vi "TWM Client Cmd Define Multiplexer Sequence.vi"(5 "timeout [ms]":i32=5000, 7 "end of packet key":string="TWM:command:EndOfPacket", 8 "error in":errorcluster, 10 "sequence item strings":string[](array[string]), 11 "handle":i32) -> (0 "error out":errorcluster, 3 "handle out":i32)   [LabVIEW 2020, in "TWM Client.lvlib"]
doc: "This will define multiplexer sequence. It's equivalent to manual setup in multiplexer panel. Sequence tag names must exist for currently selected multiplexer!"
uses:
  TWM Client.lvlib
  octave/infolib/1D String.vi
  octave/infolib/infolib.lvlib
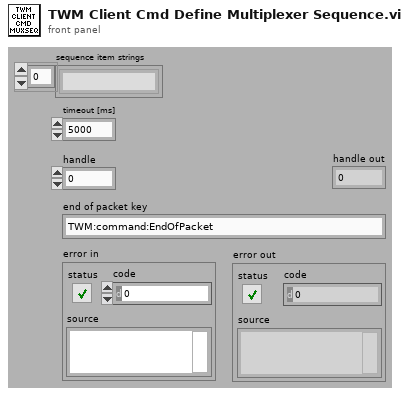
[diagram p1: front panel]
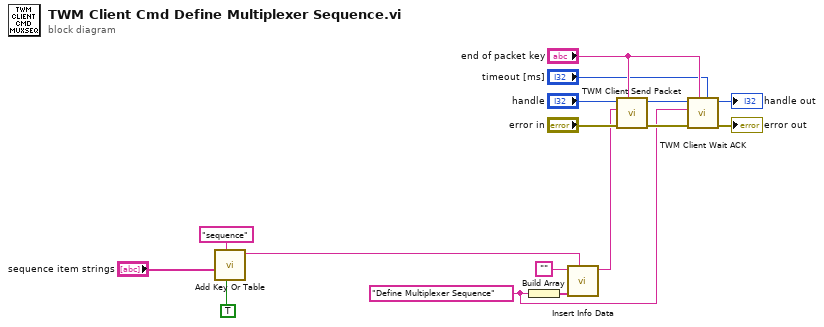
[diagram p0: block diagram]
diagram:
  w7 = "Define Multiplexer Sequence" ("section name")
  n1 = call-poly "Add Key Or Table.vi"("collumn vector (F)"=TRUE, "key description"="sequence", "string"="sequence item strings") -> ("info data out"=w1:string)  [unwired: 7 in, 1 out]
  n2 = Build Array(w7) -> (w13:string[])
  n3 = call "Insert Info Data.vi"("info data to insert"=w1, "sections"=w13, "info data"="") -> ("info data out"=w14:string)  [unwired: 7 in, 1 out]
  n4 = call "TWM Client Send Packet.vi"("end of packet key"="end of packet key", "error in"="error in", "command string"=w14, "handle"="handle") -> ("error out"=w9:errorcluster, "handle out"=w6:i32)  [unwired: 6 in]
  n5 = call "TWM Client Wait ACK.vi"("timeout [ms] (3000)"="timeout [ms]", "key string"="end of packet key", "error in"=w9, "command header"=w7, "handle"=w6) -> ("error out"=→"error out":errorcluster, "handle out"=→"handle out":i32)  [unwired: 5 in]
